vi "Sample Mean.vi"(8 "Select Data":i32=5, 9 "Technical replicate":i32, 11 "Input":string[][](array[string])) -> (0 "Sample Average":dbl[](array[numeric]), 3 "Output":string[][](array[string]))   [LabVIEW 2017]
uses:
  <vilib>/Analysis/baseanly.llb/Mean (DBL).vi
  <vilib>/Analysis/NI_AALBase.lvlib
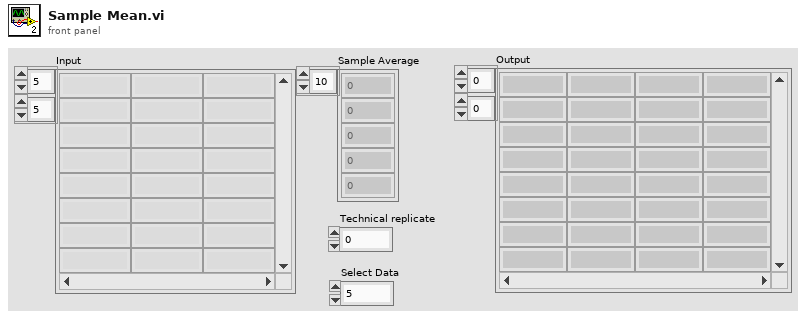
[diagram p1: front panel]
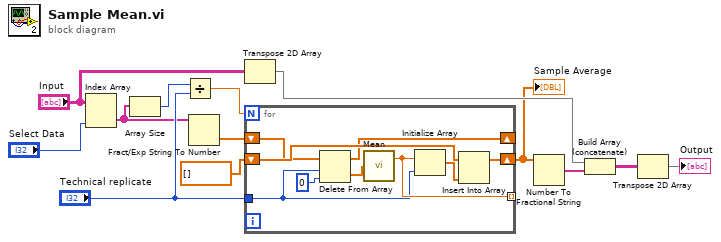
[diagram p0: block diagram]
diagram:
  n1 = Index Array(array="Input", index (col)="Select Data") -> (element=w8:string[])  [unwired: 1 in]
  n2 = Array Size(array=w8) -> (size(s)=w9:i32)
  n3 = Divide(x=w9, y="Technical replicate") -> (x/y=w10:dbl)
  n4 = Fract/Exp String To Number(string=w8) -> (number=w11:dbl[])  [unwired: 3 in, 1 out]
  n5 = Transpose 2D Array(2D array="Input") -> (transposed array=w6:string[][])
  n6 = for {
    N: w10 -> [_]
    shift-right: [w16] -> _
    shift-left: w11 -> [w15]
    tunnel: "Technical replicate" -> [w20]
    tunnel: [w21] -> _ mode=indexing
    shift-right: [w18] -> w1
    shift-left: dbl[] [] -> [w17]
    n7 = Delete From Array(array=w15, length=w20, index=0 ("인덱스")) -> (deleted portion=w14:dbl[], array with subset deleted=w16:dbl[])
    n8 = call-poly <vilib>:"Mean.vi"("X"=w14) -> ("mean"=w21:dbl)  [unwired: 1 out]
    n9 = Initialize Array(w21, w20) -> (w19:dbl[])
    n10 = Insert Into Array(array=w17, new element=w19) -> (w18:dbl[])  [unwired: 1 in]
  }
  "Sample Average" <- w1
  n11 = Number To Fractional String(number=w1) -> (F-format string=w5:string[])  [unwired: 3 in]
  n12 = Build Array (concatenate)(w6, w5) -> (w3:string[][])
  n13 = Transpose 2D Array(2D array=w3) -> (transposed array=→"Output":string[][])
